vi "LoadParam.vi"(6 "#steps":u32, 8 "error in (no error)":errorcluster, 9 "step":i32, 10 "init":i32, 11 "TelFocus in":refnum<class "TelFocus.lvclass">) -> (0 "error out":errorcluster, 3 "TelFocus out":refnum<class "TelFocus.lvclass">)   [LabVIEW 2018, in "TelFocus.lvclass"]
uses:
  TelFocus.lvclass
  TelFocus.lvclass/TelFocus.ctl
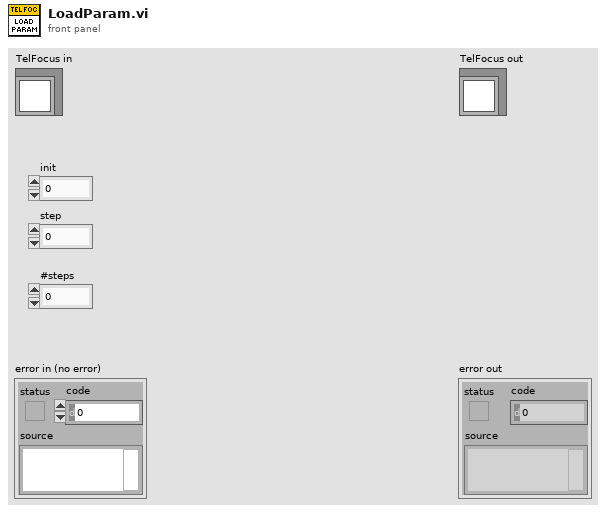
[diagram p1: front panel]
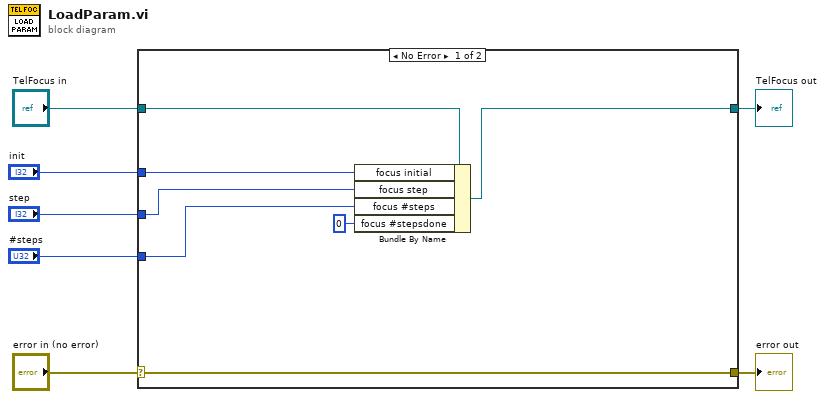
[diagram p0: block diagram]
diagram:
  n1 = case shown="No Error" "error in (no error)" {
    selector: "error in (no error)" -> [w14 w16]
    tunnel: [w14 w16] -> w6
    tunnel: [w12 w15] -> w4
    tunnel: "TelFocus in" -> [w13 w15]
    tunnel: "init" -> [w11 _]
    tunnel: "step" -> [w10 _]
    tunnel: "#steps" -> [w9 _]
    frame No Error {
      n2 = Bundle By Name(cluster=w13, "focus initial"=w11, "focus step"=w10, "focus #steps"=w9, "focus #stepsdone"=u32 0) -> (w12:refnum<class "TelFocus.lvclass">)
    }
    frame Error {
    }
  }
  "error out" <- w6
  "TelFocus out" <- w4
